vi "Performance Channel GUID.vi"() -> (3 "Performance GUID":string="1d041229-9bda-4145-b34c-c52a5f3f4f16")   [LabVIEW 2021, in "DSF Shared.lvlib"]
uses:
  DSF Shared.lvlib
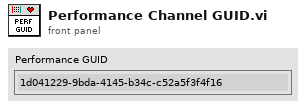
[diagram p1: front panel]
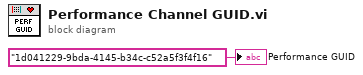
[diagram p0: block diagram]
diagram:
  "Performance GUID" <- "1d041229-9bda-4145-b34c-c52a5f3f4f16" ("Data Sharing Framework")
